vi "ProdaNG.ProductComponent.New.vi"(8 "error in (no error)":errorcluster, 10 "Product Component":T1, 11 "dbHandle":i32) -> (0 "error out":errorcluster, 3 "dbHandle":i32)   [LabVIEW 2016]
doc: "This function creates a new Product out of a prefilled product structure.\nParameter:\nhandle is an Integer, which is returned by the function Login() at the creation of a new connection.\nproduct is a pointer on a product structure, which elements must be prefilled. The structure must be defined and filled in the calling program. Nearly all elements of the structure must be set to reasonable values. The element id is filled by the DLL with a new Id for the created record, if the returncode is 0. The element crTime is being filled by the DLL automatically. The elements mdTime and mdProcessStepId are not being filled.\nThe function checks if a product with the passed WabcoPartId and serial number already exists and returns this. In this case no new product record is created.\nReturncodes:\n0 No error\n234 (ERROR_MORE_DATA) in case that the product already exists. This is no error and the product structure is returned with the existing product. \n< 0 ORACLE Error code\n6 (ERROR_INVALID_HANDLE) in case of an invalid handle"
uses:
  Controls/ProdaNG.ProductComponent.ctl
  prodllNG.dll
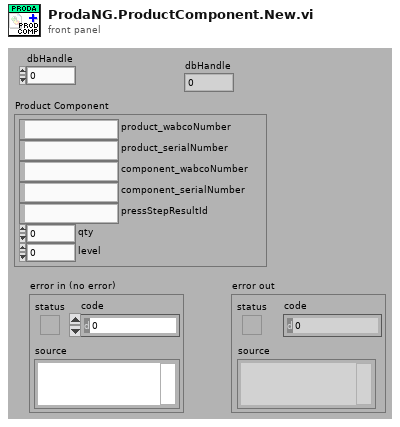
[diagram p1: front panel]
types:
  T1 = typedef "ProdaNG.ProductComponent.ctl" = cluster{"product_wabcoNumber":string, "product_serialNumber":string, "component_wabcoNumber":string, "component_serialNumber":string, "pressStepResultId":string, "qty":i32, "level":i32}
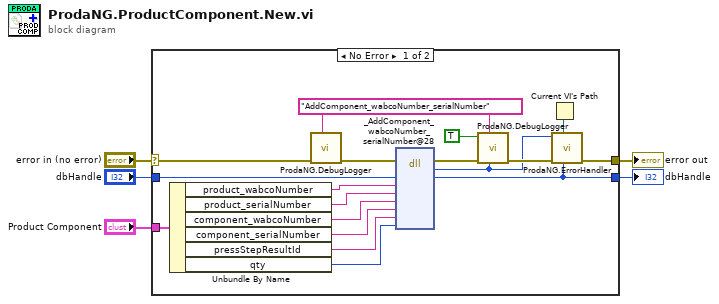
[diagram p0: block diagram]
diagram:
  n1 = case shown="No Error" "error in (no error)" {
    selector: "error in (no error)" -> [w9 w24]
    tunnel: [w22 w24] -> w4
    tunnel: "Product Component" -> [w20 _]
    tunnel: "dbHandle" -> [w18 w23]
    tunnel: [w12 w23] -> w1
    frame No Error {
      w10 = "AddComponent_wabcoNumber_serialNumber" ("cmd")
      n2 = Unbundle By Name(w20) -> ("product_wabcoNumber"=w13:string, "product_serialNumber"=w19:string, "component_wabcoNumber"=w14:string, "component_serialNumber"=w15:string, "pressStepResultId"=w16:string, "qty"=w17:i32)
      n3 = call "ProdaNG.DebugLogger.vi"("cmd"=w10, "error in (no error)"=w9) -> ("error out"=w8:errorcluster)  [unwired: 9 in]
      n4 = dll-call lib="D:/svn/LineTraceSystem/SOFTWARE/sources/Database/ProdaNG/prodllNG.dll" fn="_AddComponent_wabcoNumber_serialNumber@28" ("ProDll.dll:InitProDll")(error in=w8, "dbHandle"=w18, "product_wabcoNumber"=w13, "product_serialNumber"=w19, "component_wabcoNumber"=w14, "component_serialNumber"=w15, "processStepResultId"=w16, "qty"=w17) -> ("return type"=w6:i32, "dbHandle"=w12:i32)  [unwired: 8 in, 2 out]
      n5 = call "ProdaNG.DebugLogger.vi"("return type"=w6, "cmd"=w10, "error in (no error)"=w8, "done? (F)"=TRUE) -> ("error out"=w7:errorcluster)  [unwired: 7 in]
      n6 = Current VI's Path() -> (path=w21:path)
      n7 = call "ProdaNG.ErrorHandler.vi"("dbHandleIn"=w12, "Path"=w21, "error in"=w7, "output_parameter"=w6) -> ("error out"=w22:errorcluster)  [unwired: 7 in]
    }
    frame Error {
    }
  }
  "error out" <- w4
  "dbHandle" <- w1
